vi "ObtainPrivateQueues.vi"(8 "error in (no error)":errorcluster, 11 "DAQmx":refnum<class "DAQmx.lvclass">) -> (0 "error out":errorcluster, 3 "DAQmx out":refnum<class "DAQmx.lvclass">)   [LabVIEW 2019, in "DAQmx.lvclass"]
uses:
  DAQmx.lvclass
  typedefs/Message--Cluster.ctl
  typedefs/DAQmx.Commands--enum.ctl
  typedefs/DAQ.Config.AO--Cluster--Array.ctl
  typedefs/DAQ.Config.AO--Cluster.ctl
  typedefs/DAQ.Config.AO.Range--enum.ctl
  typedefs/DAQ.Config.Device Type--enum.ctl
  typedefs/DAQ.Config.AI--Cluster--Array.ctl
  typedefs/DAQ.Config.AI--Cluster.ctl
  typedefs/DAQ.Config.AI.Coupling--enum.ctl
  typedefs/DAQ.Config.AI.Range--enum.ctl
  typedefs/DAQ.Config.Timing--Cluster.ctl
  typedefs/DAQ.Config.Timing.Sampling--Cluster.ctl
  DAQmx.lvclass/DAQmx.ctl
panel:
  # "For instructions on how to use the JKI State Machine Objects, examples and video tutorials, visit:\nhttp://jki.net/state-machine-objects/\n\nJKI State Machine Objects™\nhttp://jki.net/state-machine-objects/\nCopyright (C) 2005-2015, JKI <info@jki.net>\nALL RIGHTS RESERVED"
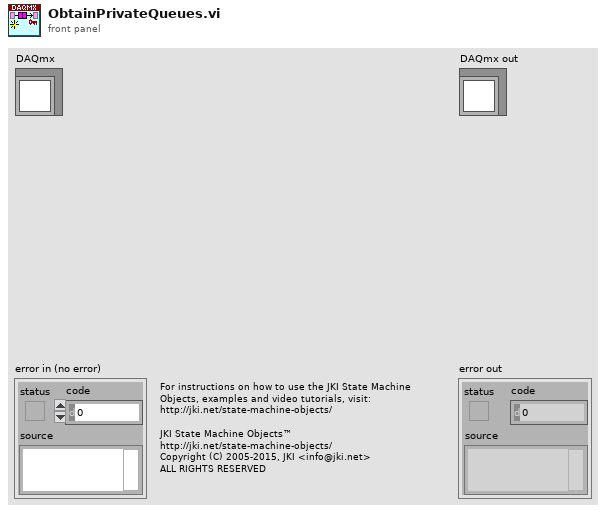
[diagram p1: front panel]
types:
  T1 = typedef "DAQmx.lvclass/Message--Cluster.ctl" = cluster{"command":T2, "Argument":string}
  T2 = typedef "DAQmx.lvclass/DAQmx.Commands--enum.ctl" = enum16{"idle", "start", "stop", "calibrate", "auto", "exit"}
  T3 = typedef "DAQmx.lvclass/DAQ.Config.AO--Cluster--Array.ctl" = T4[]
  T4 = typedef "DAQmx.lvclass/DAQ.Config.AO--Cluster.ctl" = cluster{"Channels":tag, "Range":T5, "output terminal configuration":i32, "Type":T6}
  T5 = typedef "DAQmx.lvclass/DAQ.Config.AO.Range--enum.ctl" = enum16{"±0.1", "±1.0", "±3.5", "±10.0", ""}
  T6 = typedef "DAQmx.lvclass/DAQ.Config.Device Type--enum.ctl" = enum16{"None", "USB-4431", "PXI-446x"}
  T7 = typedef "DAQmx.lvclass/DAQ.Config.AI--Cluster--Array.ctl" = T8[]
  T8 = typedef "DAQmx.lvclass/DAQ.Config.AI--Cluster.ctl" = cluster{"Channels":tag, "Coupling":T9, "Range":T10, "input terminal configuration":i32, "Type":T6}
  T9 = typedef "DAQmx.lvclass/DAQ.Config.AI.Coupling--enum.ctl" = u16
  T10 = typedef "DAQmx.lvclass/DAQ.Config.AI.Range--enum.ctl" = enum16{"±0.316", "±1.00", "±3.16", "±10.0", "±31.6", "±42.4", ""}
  T11 = typedef "DAQmx.lvclass/DAQ.Config.Timing--Cluster.ctl" = cluster{"Sampling":T12, "Fs_Out":dbl}
  T12 = typedef "DAQmx.lvclass/DAQ.Config.Timing.Sampling--Cluster.ctl" = cluster{"Fs":dbl, "#s":i32}
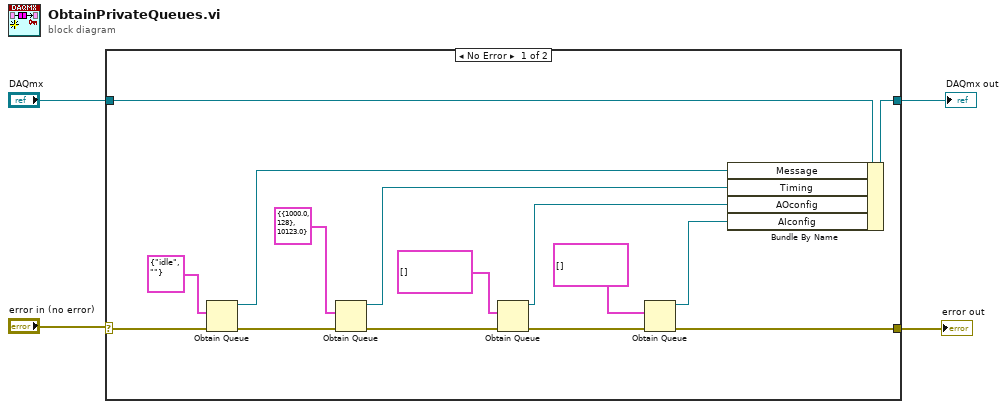
[diagram p0: block diagram]
diagram:
  n1 = case shown="No Error" "error in (no error)" {
    selector: "error in (no error)" -> [w17 w21]
    tunnel: [w9 w21] -> w2
    tunnel: [w18 w20] -> w3
    tunnel: "DAQmx" -> [w19 w20]
    frame No Error {
      n2 = Obtain Queue(element data type=T1 {"command"=enum."idle", "Argument"=""} ("Message"), error in (no error)=w17) -> (queue out=w10:refnum<queue>, error out=w16:errorcluster)  [unwired: 3 in, 1 out]
      n3 = Obtain Queue(element data type=T11 {"Sampling"={"Fs"=1000.0, "#s"=128}, "Fs_Out"=10123.0}, error in (no error)=w16) -> (queue out=w7:refnum<queue>, error out=w15:errorcluster)  [unwired: 3 in, 1 out]
      n4 = Obtain Queue(element data type=T3 [], error in (no error)=w15) -> (queue out=w6:refnum<queue>, error out=w14:errorcluster)  [unwired: 3 in, 1 out]
      n5 = Obtain Queue(element data type=T7 [], error in (no error)=w14) -> (queue out=w13:refnum<queue>, error out=w9:errorcluster)  [unwired: 3 in, 1 out]
      n6 = Bundle By Name(cluster=w19, "Message"=w10, "Timing"=w7, "AOconfig"=w6, "AIconfig"=w13) -> (w18:refnum<class "DAQmx.lvclass">)
    }
    frame Error {
    }
  }
  "error out" <- w2
  "DAQmx out" <- w3
